vi "Get Current Position Data.vi"(11 "error in":errorcluster) -> (3 "link 1 x (mm)":dbl, 4 "link 1 y (mm)":dbl, 6 "link 2 x (mm)":dbl, 10 "link 2 y (mm)":dbl, 15 "error out":errorcluster)   [LabVIEW 2017, in "myPAM.lvlib"]
uses:
  myPAM.lvlib
  Public TypeDefs/Current Position Data.ctl
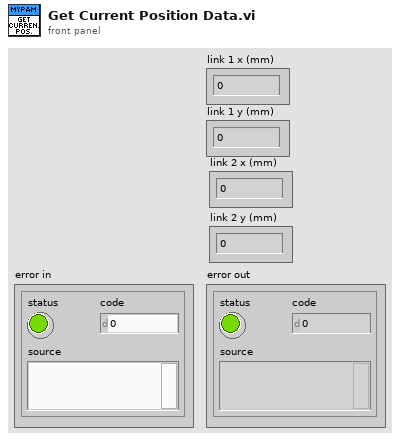
[diagram p1: front panel]
types:
  T1 = typedef "myPAM.lvlib/Current Position Data.ctl" = cluster{"link 2 x (mm)":dbl, "link 2 y (mm)":dbl, "link 1 x (mm)":dbl, "link 1 y (mm)":dbl}
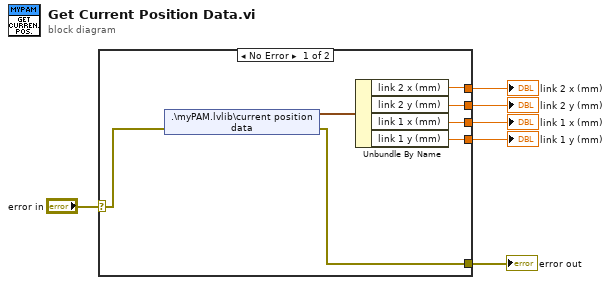
[diagram p0: block diagram]
diagram:
  n1 = case shown="No Error" "error in" {
    selector: "error in" -> [w12 w14]
    tunnel: [w11 w14] -> w5
    tunnel: [w10 _] -> w4
    tunnel: [w9 _] -> w3
    tunnel: [w8 _] -> w2
    tunnel: [w7 _] -> w1
    frame No Error {
      n2 = shared-variable ".\\myPAM.lvlib\\current position data"(error in=w12) -> (w13:T1, error out=w11:errorcluster)
      n3 = Unbundle By Name(w13) -> ("link 2 x (mm)"=w10:dbl, "link 2 y (mm)"=w9:dbl, "link 1 x (mm)"=w8:dbl, "link 1 y (mm)"=w7:dbl)
    }
    frame Error {
    }
  }
  "error out" <- w5
  "link 2 x (mm)" <- w4
  "link 2 y (mm)" <- w3
  "link 1 x (mm)" <- w2
  "link 1 y (mm)" <- w1
